vi "Messages Out_Main.vi"(8 "error in":errorcluster, 11 "QRD":T1) -> (0 "error out":errorcluster)   [LabVIEW 2025]
uses:
  Controls/Queues-Refs-Data.ctl
  Builds/Queue Wrappers.lvlibp/Q Packet.ctl
  Controls/Local Data_Messages Out.ctl
  Controls/Acquisition Packet.ctl
  Builds/Queue Wrappers.lvlibp
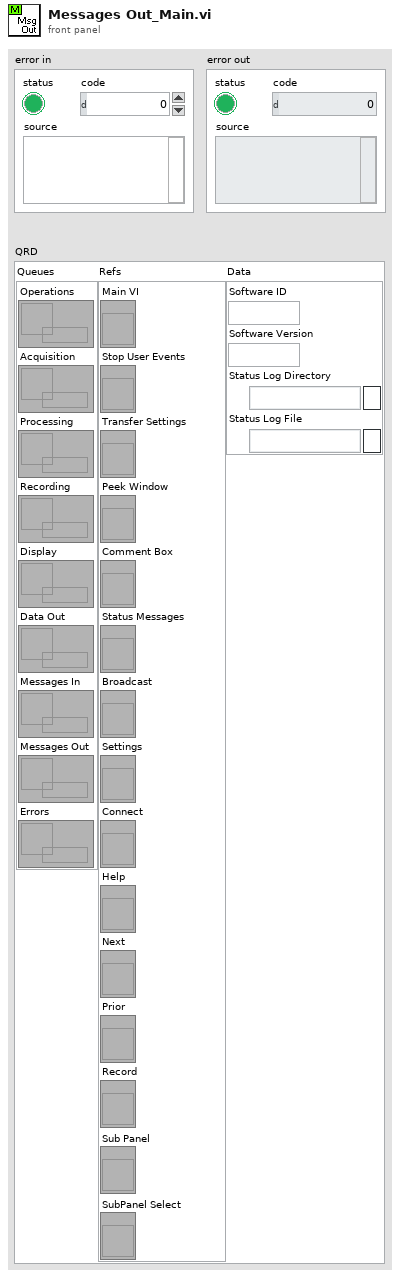
[diagram p1: front panel]
types:
  T1 = typedef "Queues-Refs-Data.ctl" = cluster{"Queues":cluster{"Operations":refnum<queue>, "Acquisition":refnum<queue>, "Processing":refnum<queue>, "Recording":refnum<queue>, "Display":refnum<queue>, "Data Out":refnum<queue>, "Messages In":refnum<queue>, "Messages Out":refnum<queue>, "Errors":refnum<queue>}, "Refs":cluster{"Main VI":refnum<vi>, "Stop User Events":refnum<vi>, "Transfer Settings":refnum<vi>, "Peek Window":refnum<vi>, "Comment Box":refnum<vi>, "Status Messages":refnum<vi>, "Broadcast":refnum<vi>, "Settings":refnum<vi>, "Connect":refnum<vi>, "Help":refnum<vi>, "Next":refnum<vi>, "Prior":refnum<vi>, "Record":refnum<vi>, "Sub Panel":refnum<vi>, "SubPanel Select":refnum<vi>}, "Data":cluster{"Software ID":string, "Software Version":string, "Status Log Directory":path, "Status Log File":path}}
  T2 = typedef "Local Data_Messages Out.ctl" = cluster{"Loop ID":string}
  T3 = typedef "Acquisition Packet.ctl" = cluster{"Time Stamp":timestamp, "Raw Data":cluster{"Instrument A":cluster{"Placeholder":string}, "Instrument B":cluster{"Placeholder":string}, "Instrument C":cluster{"Placeholder":string}}, "Derived Data":cluster{"Placeholder":string}}
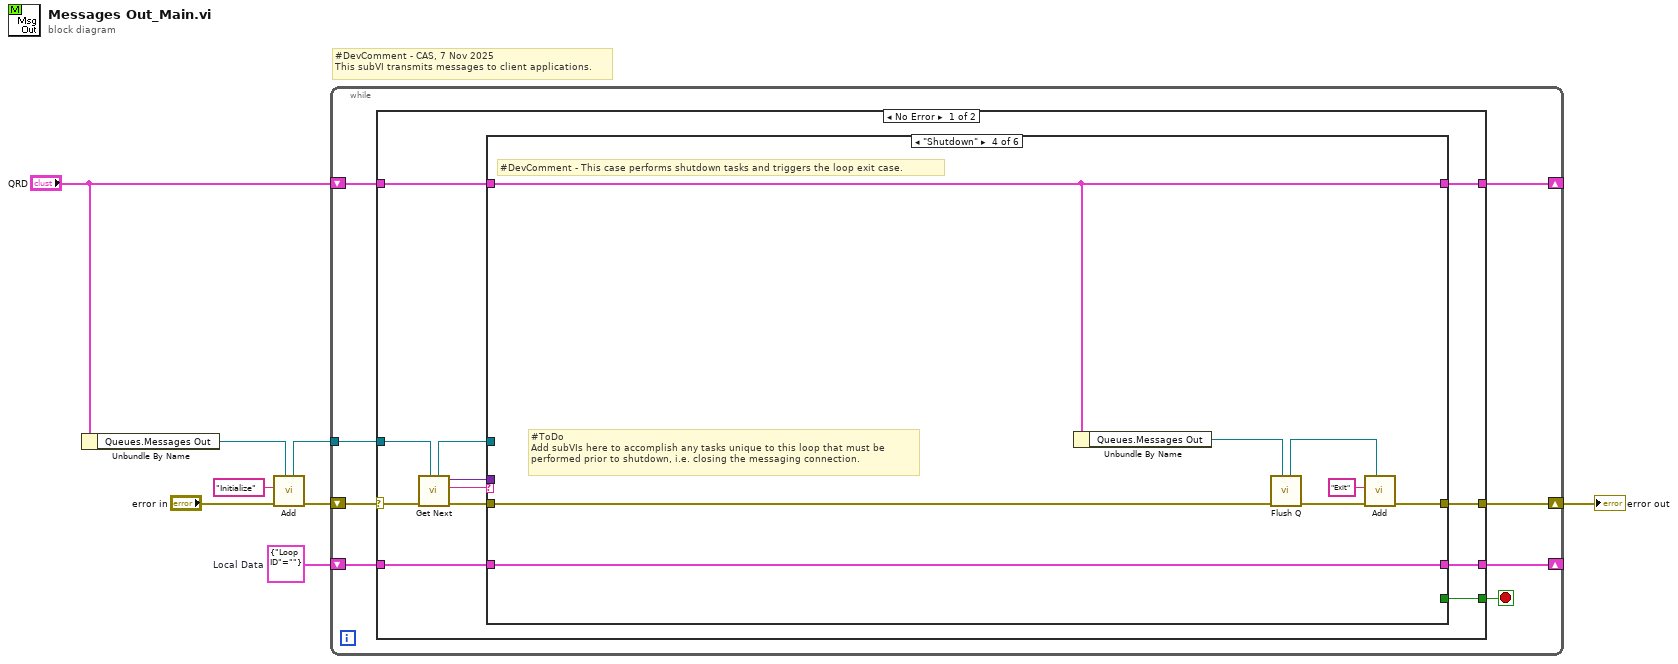
[diagram p0: block diagram]
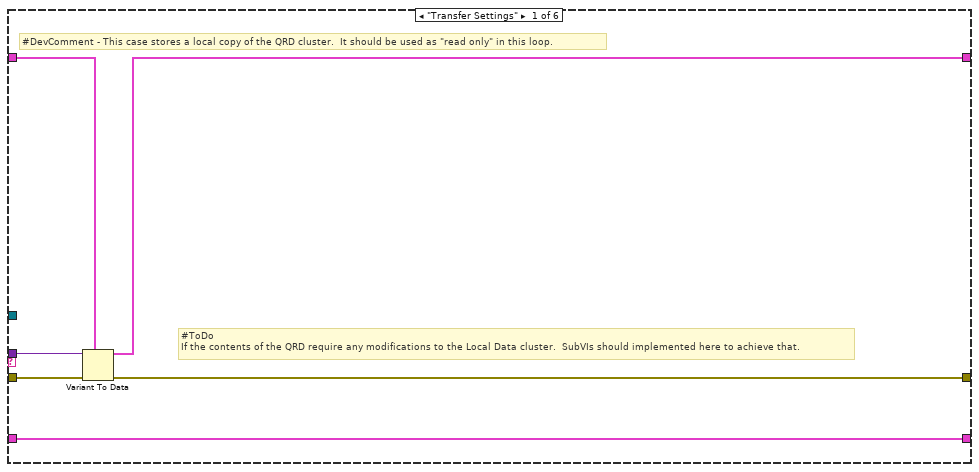
[diagram p2: hidden frame]
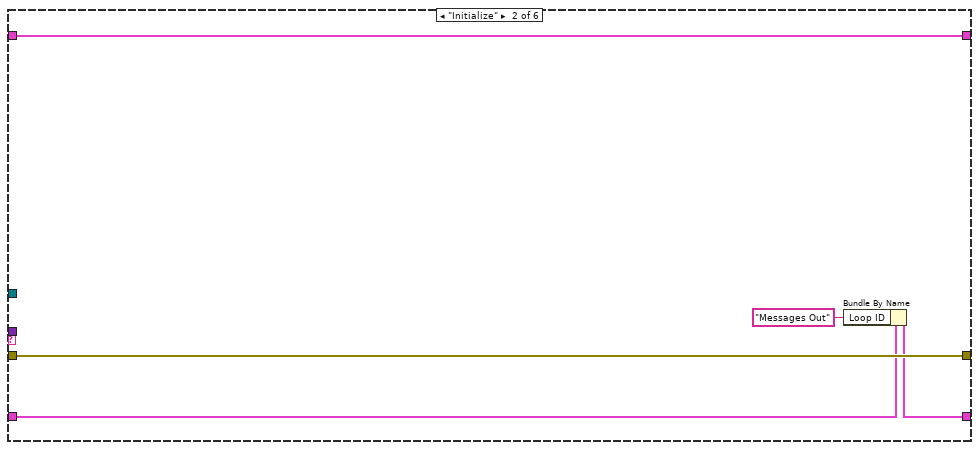
[diagram p3: hidden frame]
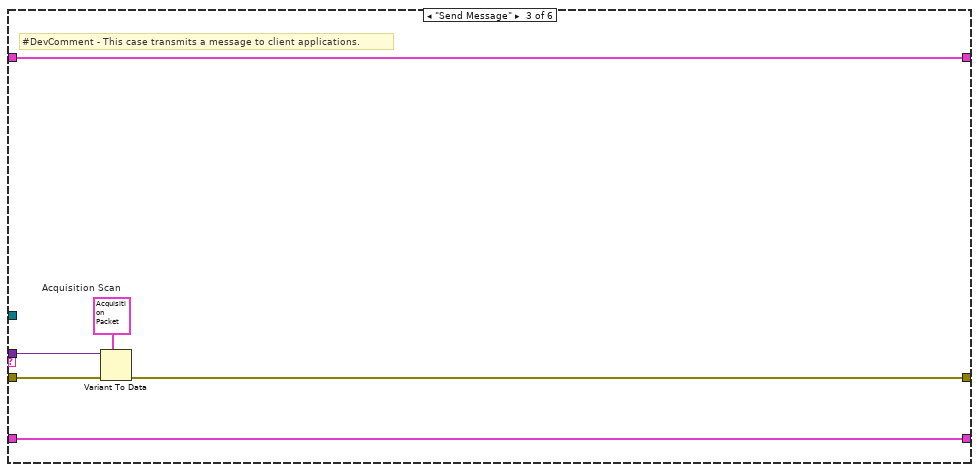
[diagram p4: hidden frame]
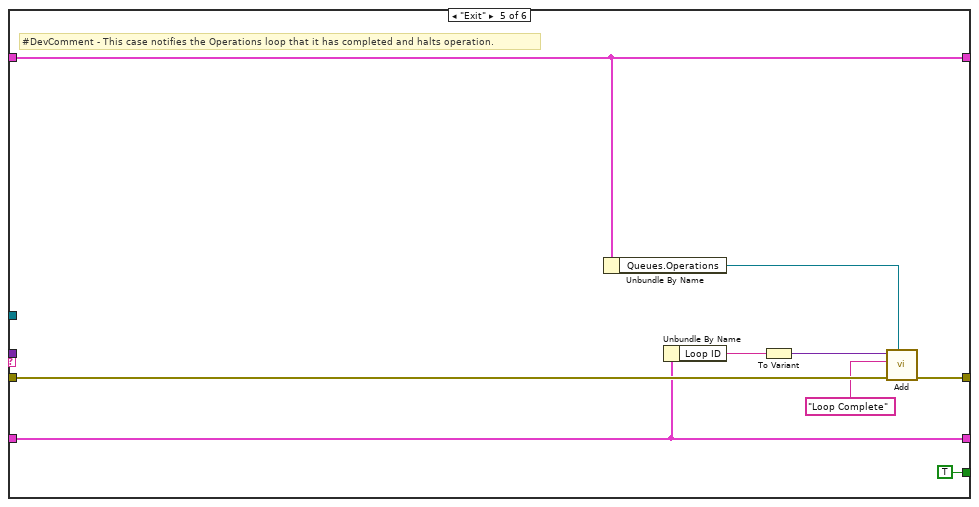
[diagram p5: hidden frame]
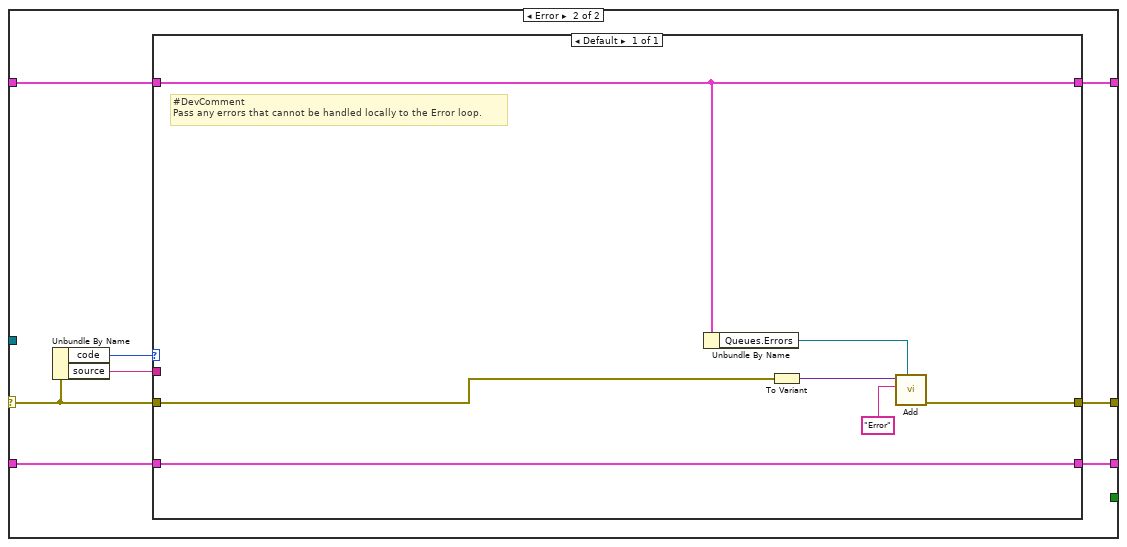
[diagram p7: hidden frame]
diagram:
  w6 = T2 {"Loop ID"=""}  # Local Data
  # "#DevComment - CAS, 7 Nov 2025\nThis subVI transmits messages to client applications."
  n1 = Unbundle By Name("QRD") -> ("Queues.Messages Out"=w3:refnum<queue>)
  n2 = call "Add.vi"("Q Ref In"=w3, "error in"="error in", "Message ID"="Initialize" ("Packet ID")) -> ("error out"=w4:errorcluster, "Q Ref Out"=w2:refnum<queue>)  [unwired: 5 in, 2 out]
  n3 = while {
    shift-right: [w15] -> _
    shift-left: "QRD" -> [w16]
    shift-right: [w13] -> w8
    shift-left: w4 -> [w14]
    tunnel: w2 -> [w12]
    shift-right: [w9] -> _
    shift-left: w6 -> [w11]
    stop <- w10 stop-if-true
    n4 = case shown="No Error" w14 {
      selector: w14 -> [w28 w70]
      tunnel: w16 -> [w25 w67]
      tunnel: [w26 w68] -> w15
      tunnel: [w23 w69] -> w13
      tunnel: w12 -> [w27 _]
      tunnel: w11 -> [w19 w71]
      tunnel: [w18 w66] -> w9
      tunnel: [w17 _] -> w10
      frame No Error {
        n5 = call "Get Next.vi"("Q Ref In"=w27, "error in"=w28) -> ("error out"=w24:errorcluster, "Message ID"=w20:string, "Payload"=w21:variant, "Q Ref Out"=w22:refnum<queue>)  [unwired: 6 in]
        n6 = case shown="\"Shutdown\"" w20 {
          tunnel: [w30 w39 w40 w53 w62 w65] -> w26
          tunnel: w25 -> [w32 w39 w40 w53 w62 w65]
          tunnel: w24 -> [w34 w38 w45 w51 w60 w64]
          tunnel: [w31 w38 w42 w52 w61 w64] -> w23
          tunnel: w22 -> [_ _ _ _ _ _]
          tunnel: w21 -> [w33 _ w44 _ _ _]
          tunnel: w19 -> [w29 w36 w41 w47 w58 w63]
          tunnel: [w29 w37 w41 w47 w58 w63] -> w18
          tunnel: [_ _ _ _ TRUE _] -> w17
          frame "Transfer Settings" {
            # "#ToDo\nIf the contents of the QRD require any modifications to the Local Data cluster.  SubVIs should implemented here to achieve that."
            # "#DevComment - This case stores a local copy of the QRD cluster.  It should be used as \"read only\" in this loop."
            n7 = Variant To Data(error in=w34, type=w32, Variant=w33) -> (data=w30:T1, error out=w31:errorcluster)
          }
          frame "Initialize" {
            n8 = Bundle By Name(cluster=w36, "Loop ID"="Messages Out") -> (w37:T2)
          }
          frame "Send Message" {
            w43 = T3 {"Time Stamp"=timestamp(0 s since 1904-01-01), "Raw Data"={"Instrument A"={"Placeholder"=""}, "Instrument B"={"Placeholder"=""}, "Instrument C"={"Placeholder"=""}}, "Derived Data"={"Placeholder"=""}}  # Acquisition Scan
            # "#DevComment - This case transmits a message to client applications."
            n9 = Variant To Data(error in=w45, type=w43, Variant=w44) -> (error out=w42:errorcluster)  [unwired: 1 out]
          }
          frame "Shutdown" {
            # "#ToDo\nAdd subVIs here to accomplish any tasks unique to this loop that must be\nperformed prior to shutdown, i.e. closing the messaging connection."
            # "#DevComment - This case performs shutdown tasks and triggers the loop exit case."
            n10 = Unbundle By Name(w53) -> ("Queues.Messages Out"=w49:refnum<queue>)
            n11 = call "Flush Q.vi"("Q Ref In"=w49, "error in"=w51) -> ("error out"=w50:errorcluster, "Q Ref Out"=w48:refnum<queue>)  [unwired: 7 in, 1 out]
            n12 = call "Add.vi"("Q Ref In"=w48, "error in"=w50, "Message ID"="Exit" ("Packet ID")) -> ("error out"=w52:errorcluster)  [unwired: 5 in, 3 out]
          }
          frame "Exit" {
            # "#DevComment - This case notifies the Operations loop that it has completed and halts operation."
            n13 = Unbundle By Name(w62) -> ("Queues.Operations"=w59:refnum<queue>)
            n14 = Unbundle By Name(w58) -> ("Loop ID"=w57:string)
            n15 = To Variant(anything=w57) -> (Variant=w54:variant)
            n16 = call "Add.vi"("Q Ref In"=w59, "error in"=w60, "Message ID"="Loop Complete" ("Packet ID"), "Payload"=w54) -> ("error out"=w61:errorcluster)  [unwired: 4 in, 3 out]
          }
          frame Default {
          }
        }
      }
      frame Error {
        n17 = Unbundle By Name(w70) -> ("code"=w73:i32, "source"=w72:string)
        n18 = case shown="Default" w73 {
          tunnel: w72 -> [_]
          tunnel: w71 -> [w80]
          tunnel: [w80] -> w66
          tunnel: w70 -> [w76]
          tunnel: [w78] -> w69
          tunnel: [w77] -> w68
          tunnel: w67 -> [w77]
          frame Default {
            # "#DevComment\nPass any errors that cannot be handled locally to the Error loop."
            n19 = Unbundle By Name(w77) -> ("Queues.Errors"=w79:refnum<queue>)
            n20 = To Variant(anything=w76) -> (Variant=w74:variant)
            n21 = call "Add.vi"("Q Ref In"=w79, "Message ID"="Error" ("Packet ID"), "Payload"=w74) -> ("error out"=w78:errorcluster)  [unwired: 5 in, 3 out]
          }
        }
      }
    }
  }
  "error out" <- w8
